vi "Tree.vi"   [LabVIEW 2019, in "JSON-Schema.lvlib"]
uses:
  JSON-Schema.lvlib
  API/Read Typedef Description (variant).vi
  API/Write Typedef Description (variant).vi
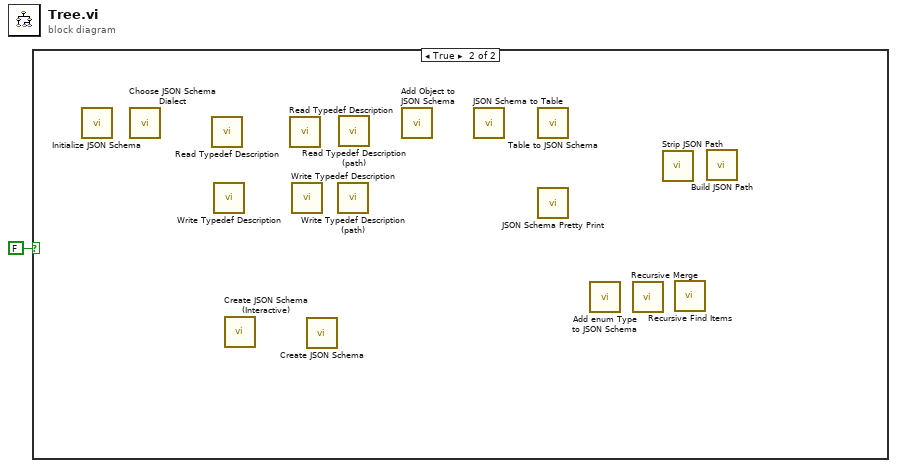
[diagram p0: block diagram]
diagram:
  n1 = case shown="True" FALSE {
    frame False {
    }
    frame True {
      n2 = call "Initialize JSON Schema.vi"() -> ()  [unwired: 10 in, 2 out]
      n3 = call "Choose JSON Schema Dialect.vi"() -> ()  [unwired: 10 in, 2 out]
      n4 = call-poly "Read Typedef Description.vi"() -> ()  [unwired: 9 in, 3 out]
      n5 = call-poly "Write Typedef Description.vi"() -> ()  [unwired: 10 in, 2 out]
      n6 = call "Create JSON Schema (Interactive).vi"() -> ()  [unwired: 10 in, 2 out]
      n7 = call-poly "Read Typedef Description.vi"() -> ()  [unwired: 9 in, 3 out]
      n8 = call-poly "Write Typedef Description.vi"() -> ()  [unwired: 10 in, 2 out]
      n9 = call "Create JSON Schema.vi"() -> ()  [unwired: 11 in, 1 out]
      n10 = call "Write Typedef Description (path).vi"() -> ()  [unwired: 10 in, 2 out]
      n11 = call "Read Typedef Description (path).vi"() -> ()  [unwired: 9 in, 3 out]
      n12 = call "Add Object to JSON Schema.vi"() -> ()  [unwired: 8 in, 4 out]
      n13 = call "JSON Schema to Table.vi"() -> ()  [unwired: 9 in, 3 out]
      n14 = call "Table to JSON Schema.vi"() -> ()  [unwired: 10 in, 2 out]
      n15 = call "JSON Schema Pretty Print.vi"() -> ()  [unwired: 10 in, 2 out]
      n16 = call "Add enum Type to JSON Schema.vi"() -> ()  [unwired: 10 in, 2 out]
      n17 = call "Recursive Merge.vi"() -> ()  [unwired: 10 in, 2 out]
      n18 = call "Strip JSON Path.vi"() -> ()  [unwired: 9 in, 3 out]
      n19 = call "Recursive Find Items.vi"() -> ()  [unwired: 8 in, 4 out]
      n20 = call "Build JSON Path.vi"() -> ()  [unwired: 11 in, 1 out]
    }
  }
